vi "Prober_ReadXYZTheta.vi"(8 "error in (no error)":errorcluster, 11 "ProbeStationControl in":refnum<class "ProbeStationControl.lvclass">) -> (0 "error out":errorcluster, 1 "Z location [µm]":i32, 2 "Y location [µm]":i32, 3 "X location [µm]":i32, 4 "Theta location [mdeg]":i32, 5 "ProbeStationControl out":refnum<class "ProbeStationControl.lvclass">)   [LabVIEW 2019, in "ProbeStationControl.lvclass"]
uses:
  ProbeStationControl.lvclass
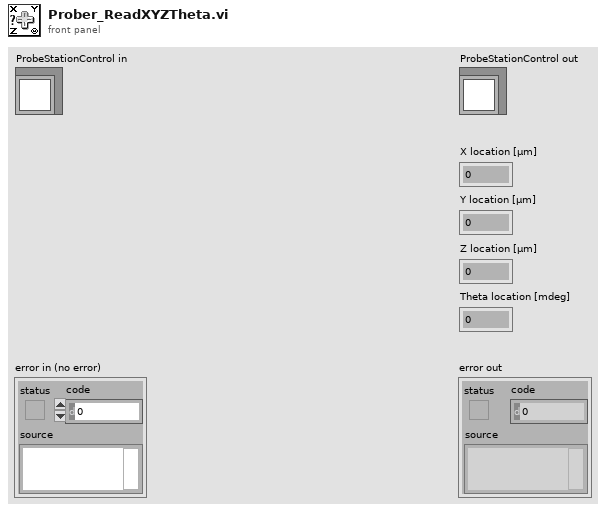
[diagram p1: front panel]
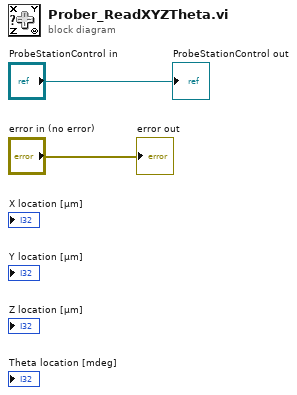
[diagram p0: block diagram]
diagram:
  "error out" <- "error in (no error)"
  "ProbeStationControl out" <- "ProbeStationControl in"
